vi "Configure Period.vi"(8 "error in (no error)":errorcluster, 9 "Period (seconds)":dbl=0.01 min=0.01 max=9999.0 step=0.01, 10 "Memory":u32(ring) items=["Not Available", "Available"], 11 "VISA resource name":refnum<visa-resource-name>) -> (0 "error out":errorcluster, 3 "VISA resource name out":refnum<visa-resource-name>)   [LabVIEW 2022 SP3, in "MagnaDC.lvlib"]
uses:
  MagnaDC.lvlib
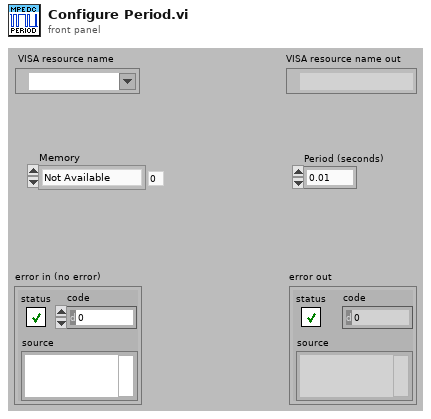
[diagram p1: front panel]
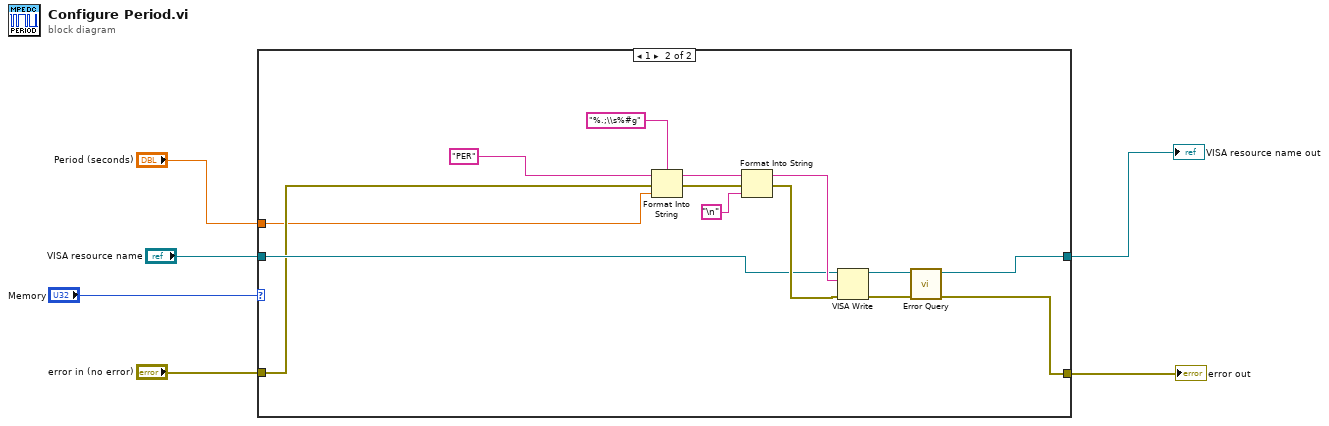
[diagram p0: block diagram]
diagram:
  n1 = case shown="1" "Memory" {
    tunnel: "VISA resource name" -> [w8 w13]
    tunnel: [w8 w12] -> w4
    tunnel: "error in (no error)" -> [w7 w10]
    tunnel: [w7 w11] -> w2
    tunnel: "Period (seconds)" -> [_ w9]
    frame 0, Default {
    }
    frame 1 {
      n2 = Format Into String(format string="%.;\\s%#g", initial string="PER", error in=w10, w9) -> (resulting string=w22:string, error out=w21:errorcluster)
      n3 = Format Into String(initial string=w22, error in=w21, "\n") -> (resulting string=w19:string, error out=w20:errorcluster)  [unwired: 1 in]
      n4 = VISA Write(VISA resource name=w13, write buffer=w19, error in (no error)=w20) -> (VISA resource name out=w17:refnum<visa-resource-name>, error out=w18:errorcluster)  [unwired: 1 out]
      n5 = call "Error Query.vi"("error in (no error)"=w18, "VISA resource name"=w17) -> ("error out"=w11:errorcluster, "VISA resource name out"=w12:refnum<visa-resource-name>)  [unwired: 6 in, 2 out]
    }
  }
  "error out" <- w2
  "VISA resource name out" <- w4
